vi "ATF-Pump-DI Data FGV.vi"(8 "DI Y LP":bool[](array[boolean]), 9 "DI LOX-LP data":digitalwaveform[](array[waveform]), 10 "DI Signal List LP":string[](array[string]), 11 "Write/Read":T1=enum."Read") -> (0 "DI Y LP":bool[](array[boolean]), 1 "DI LOX-LP data":digitalwaveform[](array[waveform]), 2 "DI Signal List LP":string[](array[string]))   [LabVIEW 2022 SP3]
uses:
  RT Controls/ATF-Pump-FGV Read write.ctl
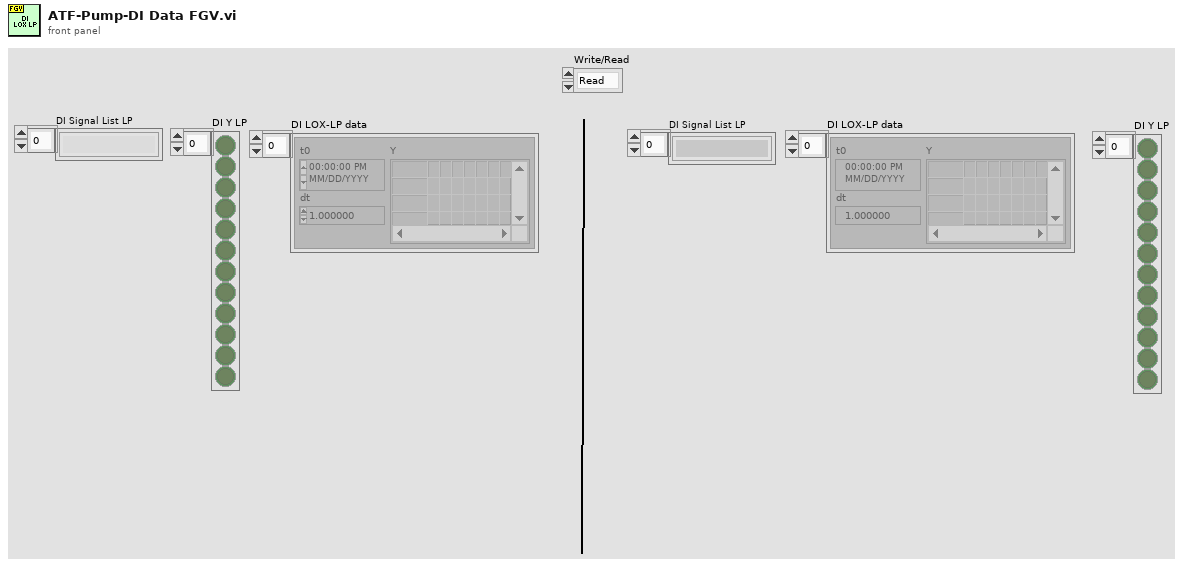
[diagram p1: front panel]
types:
  T1 = typedef "ATF-Pump-FGV Read write.ctl" = enum16{"Write", "Read"}
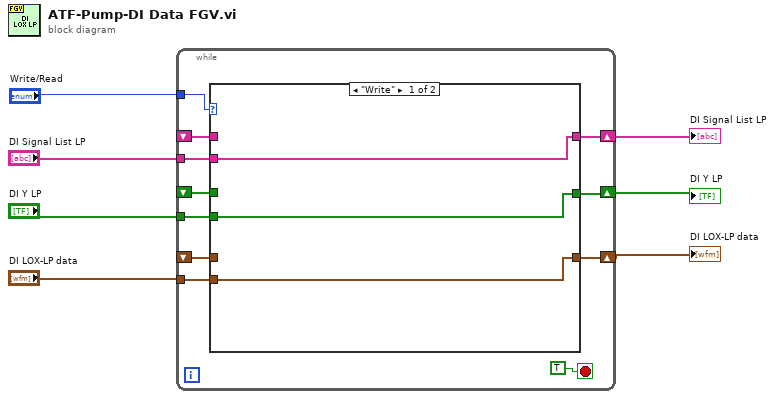
[diagram p0: block diagram]
diagram:
  n1 = while {
    tunnel: "Write/Read" -> [w17]
    shift-right: [w16] -> w7
    shift-left: _ -> [w15]
    shift-right: [w14] -> w2
    shift-left: _ -> [w13]
    shift-right: [w12] -> w4
    shift-left: _ -> [w11]
    tunnel: "DI Signal List LP" -> [w10]
    tunnel: "DI Y LP" -> [w9]
    tunnel: "DI LOX-LP data" -> [w8]
    stop <- TRUE stop-if-true
    n2 = case shown="\"Write\"" w17 {
      tunnel: [w21 w24] -> w16
      tunnel: w15 -> [_ w24]
      tunnel: [w20 w23] -> w14
      tunnel: w13 -> [_ w23]
      tunnel: [w19 w22] -> w12
      tunnel: w11 -> [_ w22]
      tunnel: w10 -> [w21 _]
      tunnel: w9 -> [w20 _]
      tunnel: w8 -> [w19 _]
      frame "Write" {
      }
      frame "Read" {
      }
    }
  }
  "DI Signal List LP" <- w7
  "DI LOX-LP data" <- w4
  "DI Y LP" <- w2
